vi "daq_thermistors.vi"(1 "Timeout":i32) -> (0 "FIFO_timeout":bool)   [LabVIEW 2018]
uses:
  <vilib>/rvi/eio/common/nirviEmuTemplateMethod_errors.vi
  <vilib>/rvi/DataTransferAndStorage/Container/Common/niFpgaContainerExecOnDevCompGetState.vi
  <vilib>/rvi/Emulation/niFpgaEmulationIsFPGAContextNoSignature.vi
  <vilib>/rvi/Emulation/niFpgaSctlEmulationGetInTimedLoop.vi
  <vilib>/rvi/errors/niFpgaSetErrorForExecOnDevCompSimple.vi
  <vilib>/rvi/eio/common/nirviEmuReportErrorAndStop.vi
  <vilib>/rvi/DataTransferAndStorage/Container/Common/niFpgaContainerGetUniqueNameForEmu.vi
  <vilib>/rvi/FIFO/Fifo_Resource/nirvififoEmulationSetSize.vi
  <vilib>/rvi/FIFO/Fifo_Resource/nirviFifoEmulationQueueMgr.vi
  <instcachedir>/0/nirviFifoEmulationQueueMgr_E5CAEC123FF24DC58D834DCA3CDAA9B5.lvgen/nirviFifoEmulationQueueMgr_E5CAEC123FF24DC58D834DCA3CDAA9B5_002.vi
  <vilib>/rvi/FIFO/Fifo_Resource/nirvififoEmulationDetermineInputValidOut.vi
  <vilib>/rvi/FIFO/Fifo_Resource/nirvififoEmulationCreateLock.vi
  <vilib>/rvi/Emulation/niFpgaProcessEmulError.vi
  <vilib>/rvi/FIFO/Fifo_Resource/nirvififoEmulationObtainLock.vi
  <vilib>/rvi/FIFO/Fifo_Resource/nirvififoEmulationReleaseLock.vi
  <vilib>/rvi/occurrence/nirviWaitOnOccurrenceBase.vi
  <vilib>/rvi/errors/nirviReportUnexpectedCaseInternalError.vi
  <vilib>/rvi/errors/nirviReportUnexpectedCaseInternalError (U32).vi
  <vilib>/Utility/error.llb/Clear Errors.vi
  <vilib>/rvi/interface/RandomDataEmulation/niFpgaRandomDataHandleErrors.vi
  <vilib>/eio/EIONode/EIONode.xnode
  <vilib>/rvi/DataTransferAndStorage/Container/XNode/niFpgaContainer.xnode
  <vilib>/rvi/FIFO/Fifo_Resource/niFpgaFifoEmulationRefIn.vi
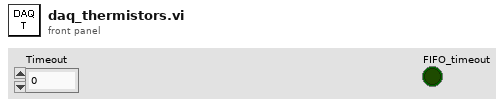
[diagram p1: front panel]
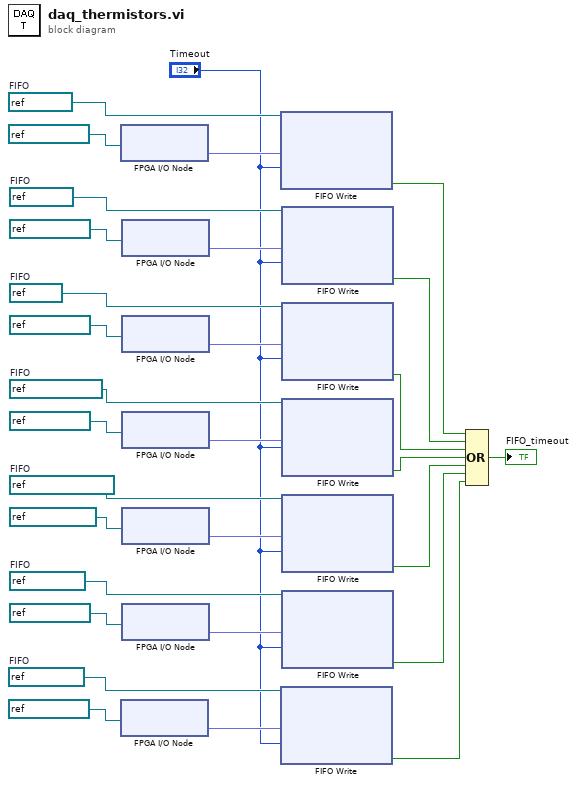
[diagram p0: block diagram]
diagram:
  w5 = refnum<k21> "T_extra_2"  # FIFO
  w14 = refnum<k21> "T_extra_1"  # FIFO
  w17 = refnum<k21> "T_pneum_tank"  # FIFO
  w20 = refnum<k21> "T_pod_temp"  # FIFO
  w23 = refnum<k21> "T_RB"  # FIFO
  w26 = refnum<k21> "T_PB_2"  # FIFO
  w29 = refnum<k21> "T_PB_1"  # FIFO
  n1 = xnode "FPGA I/O Node"("FPGA I/O In"=refnum<k21> "Mod1/AI6") -> ("I/O Item"=w28:fxp<+/-,24,5>)  [unwired: 1 out]
  n2 = xnode "FPGA I/O Node"("FPGA I/O In"=refnum<k21> "Mod1/AI3") -> ("I/O Item"=w4:fxp<+/-,24,5>)  [unwired: 1 out]
  n3 = xnode "FPGA I/O Node"("FPGA I/O In"=refnum<k21> "Mod1/AI7") -> ("I/O Item"=w25:fxp<+/-,24,5>)  [unwired: 1 out]
  n4 = xnode "FPGA I/O Node"("FPGA I/O In"=refnum<k21> "Mod1/AI8") -> ("I/O Item"=w22:fxp<+/-,24,5>)  [unwired: 1 out]
  n5 = xnode "FPGA I/O Node"("FPGA I/O In"=refnum<k21> "Mod1/AI9") -> ("I/O Item"=w19:fxp<+/-,24,5>)  [unwired: 1 out]
  n6 = xnode "FPGA I/O Node"("FPGA I/O In"=refnum<k21> "Mod1/AI10") -> ("I/O Item"=w16:fxp<+/-,24,5>)  [unwired: 1 out]
  n7 = xnode "FPGA I/O Node"("FPGA I/O In"=refnum<k21> "Mod1/AI2") -> ("I/O Item"=w13:fxp<+/-,24,5>)  [unwired: 1 out]
  n8 = xnode "FIFO Write"("Element"=w28, "Timeout"="Timeout", "FIFO In"=w29) -> ("Timed Out?"=w12:bool)  [unwired: 1 out]
  n9 = xnode "FIFO Write"("Element"=w4, "Timeout"="Timeout", "FIFO In"=w5) -> ("Timed Out?"=w2:bool)  [unwired: 1 out]
  n10 = xnode "FIFO Write"("Element"=w25, "Timeout"="Timeout", "FIFO In"=w26) -> ("Timed Out?"=w11:bool)  [unwired: 1 out]
  n11 = xnode "FIFO Write"("Element"=w22, "Timeout"="Timeout", "FIFO In"=w23) -> ("Timed Out?"=w10:bool)  [unwired: 1 out]
  n12 = xnode "FIFO Write"("Element"=w19, "Timeout"="Timeout", "FIFO In"=w20) -> ("Timed Out?"=w8:bool)  [unwired: 1 out]
  n13 = xnode "FIFO Write"("Element"=w16, "Timeout"="Timeout", "FIFO In"=w17) -> ("Timed Out?"=w9:bool)  [unwired: 1 out]
  n14 = xnode "FIFO Write"("Element"=w13, "Timeout"="Timeout", "FIFO In"=w14) -> ("Timed Out?"=w1:bool)  [unwired: 1 out]
  n15 = Compound Arithmetic op=OR(w12, w11, w10, w8, w9, w1, w2) -> (→"FIFO_timeout":bool)
